vi "upload.sign_part.vi"(6 "Part Number":i32, 8 "error in":errorcluster, 11 "Multipart Upload in":refnum<class "Multipart Upload.lvclass">) -> (0 "error out":errorcluster, 3 "Multipart Upload out":refnum<class "Multipart Upload.lvclass">)   [LabVIEW 2020, in "Multipart Upload.lvclass"]
doc: "Signs an upload request for a single part. Returns a URL that will execute the upload without further authentication.\n\nThe Part Number must be greater than 0."
uses:
  Nominal Client MultiPart Upload/Multipart Upload.lvclass
  Nominal Client MultiPart Upload/Multipart Upload.lvclass/Multipart Upload.ctl
  8b3dcdab-c30a-41f7-882b-0fd92512159b.vi
  Nominal Client MultiPart Upload/nominal_client.get.vi
  <vilib>/JDP Science/JSONtext/JSON text to Variant.vi
  Nominal Client.lvclass
  <vilib>/JDP Science/JSONtext/LVClass Serializer/JSONtext LVClass Serializer.lvclass
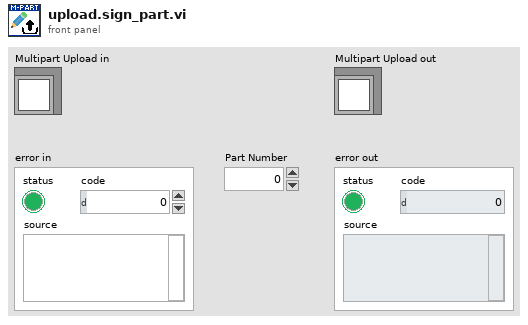
[diagram p1: front panel]
types:
  T1 = map{i32, cluster{"url":string, "headers":string}}
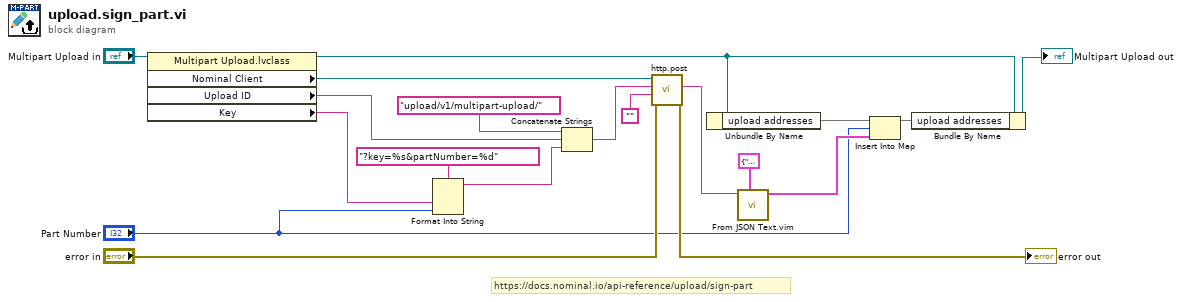
[diagram p0: block diagram]
diagram:
  # "https://docs.nominal.io/api-reference/upload/sign-part"
  n1 = property class="Multipart Upload.lvclass"(reference="Multipart Upload in") -> (reference out=w3:refnum<class "Multipart Upload.lvclass">, "Nominal Client"=w7:refnum<class "Nominal Client.lvclass">, "Upload ID"=w10:string, "Key"=w9:string)  [unwired: 1 in, 1 out]
  n2 = Format Into String(format string="?key=%s&partNumber=%d" ("Path"), w9, "Part Number") -> (resulting string=w12:string)  [unwired: 2 in, 1 out]
  n3 = Concatenate Strings("upload/v1/multipart-upload/" ("Path"), w10, w12) -> (w15:string)
  n4 = call "http.post.vi"("error in"="error in", "Request body"="", "Path"=w15, "Nominal Client in"=w7) -> ("error out"=→"error out":errorcluster, "Response"=w17:string)  [unwired: 4 in, 2 out]
  n5 = Unbundle By Name(w3) -> ("upload addresses"=w6:T1)
  n6 = call "From JSON Text.vim"("Data Type and Default Value"=cluster{"url":string, "headers":string} {"url"="", "headers"=""}, "JSON"=w17) -> ("Data out"=w5:cluster{"url":string, "headers":string})  [unwired: 8 in, 1 out]
  n7 = Insert Into Map(map in=w6, key="Part Number", value=w5) -> (map out=w1:T1)  [unwired: 2 out]
  n8 = Bundle By Name(cluster=w3, "upload addresses"=w1) -> (→"Multipart Upload out":refnum<class "Multipart Upload.lvclass">)
